vi "写入颜色.vi"(8 "error in (no error)":errorcluster caption="错误输入（无错误）", 10 "颜色":u32(colorbox), 11 "点输入":refnum<class "点.lvclass">) -> (0 "error out":errorcluster caption="错误输出", 3 "点输出":refnum<class "点.lvclass">)   [LabVIEW 2011]
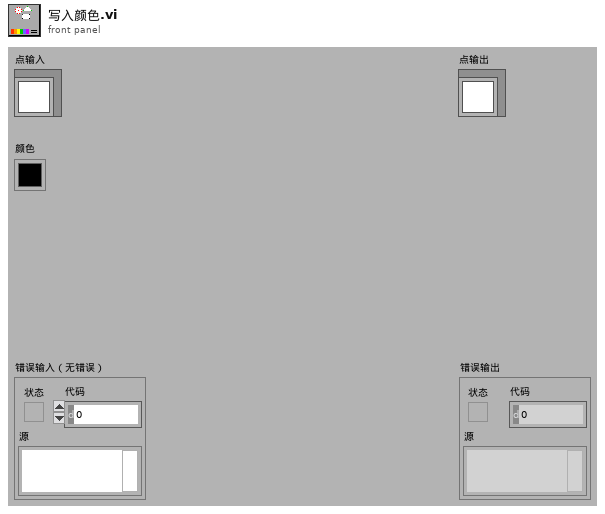
[diagram p1: front panel]
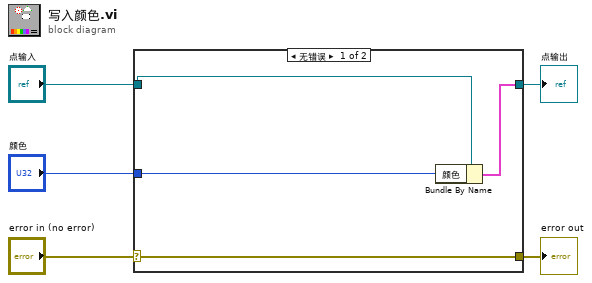
[diagram p0: block diagram]
diagram:
  n1 = case shown="无错误" "error in (no error)" {
    selector: "error in (no error)" -> [w9 w10]
    tunnel: [w9 w10] -> w4
    tunnel: [w7 w11] -> w2
    tunnel: "点输入" -> [w8 w11]
    tunnel: "颜色" -> [w6 _]
    frame No Error {
      n2 = Bundle By Name(cluster=w8, "颜色"=w6) -> (w7:cluster{})
    }
    frame Error {
    }
  }
  "error out" <- w4
  "点输出" <- w2
